vi "AlliGator Build Image Profile Plots.vi"(0 "Intensity":dbl[](array[numeric]), 1 "ROI Type":T4, 2 "Box Profile Type":T3, 3 "ROI Size String":string, 5 "Phase Lifetime":dbl[](array[numeric]), 7 "Average Lifetime/Phasor Ratio":dbl[](array[numeric]), 9 "Fit Parameter":dbl[](array[numeric]), 11 "Error In":errorcluster, 12 "Fit Parameter Name":string, 13 "ratio(T)/<tau>(F)":bool, 14 "< t>_I (F)/<t>_A":bool) -> (4 "Plot Array":T1[](array[typedef]), 15 "Error Out":errorcluster)   [LabVIEW 2021, in "AlliGator Image Profile Window.lvlib"]
doc: "Builds the array of displayed profiles according to the user-selected options and ROI type."
uses:
  AlliGator Image Profile Window.lvlib
  Image/Image ROI Type.ctl
  Image/Box Profile Type.ctl
  AlliGator Image Profile Plot Data.ctl
  Graphs/XY Graph/XY Plot Data.ctl
  Arrays/Linear Ramp End Options.ctl
  52adedef-4fce-46da-a191-00be4efc5a4e.vi
  7c534c3e-da10-41db-a8ff-5ea6a11f1b7c.vi
  c62035f1-53a3-4edf-964a-62b160a8d83f.vi
  258de3ba-5316-44aa-b6b1-8f05b3134f67.vi
  Graphs/XY Graph/XY Graph Add-Ons.lvlib
  Arrays/Arrays.lvlib
  Image/Image.lvlib
panel:
  # "see the AlliGator License on the block diagram (Ctrl+E or Window:Show Block Diagram)"
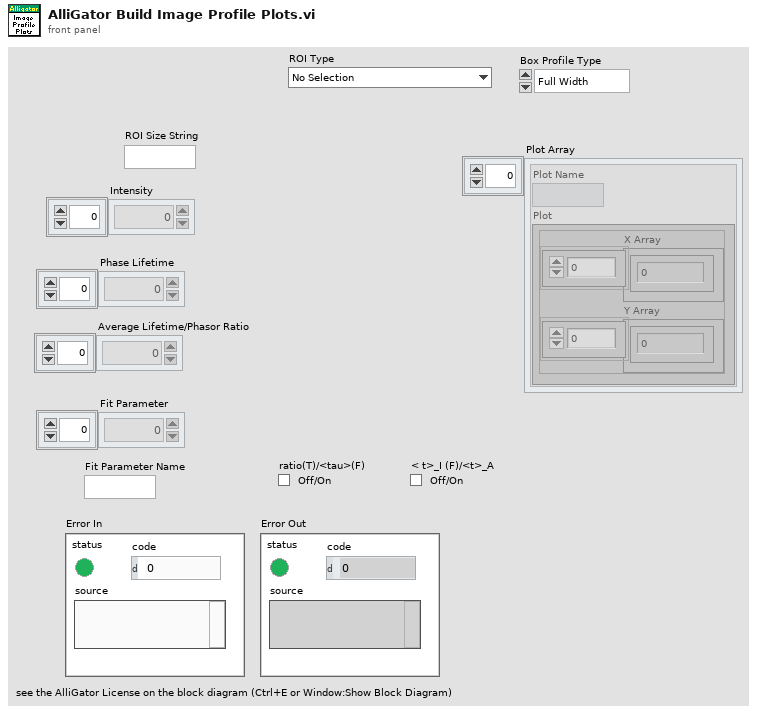
[diagram p1: front panel]
types:
  T1 = typedef "AlliGator Image Profile Window.lvlib/AlliGator Image Profile Plot Data.ctl" = cluster{"Plot Name":string, "Plot":T2}
  T2 = typedef "XY Graph Add-Ons.lvlib/XY Plot Data.ctl" = cluster{"X Array":dbl[], "Y Array":dbl[]}
  T3 = typedef "Image.lvlib/Box Profile Type.ctl" = enum16{"Full Width", "Half Width"}
  T4 = typedef "Image.lvlib/Image ROI Type.ctl" = enum16{"No Selection", "Point", "Line", "Rectangle", "Oval", "Polygon", "Freehand Region", "Annulus", "Unused2", "Unused3", "Broken Line", "Freehand Line", "Rotated Rectangle"}
  T5 = typedef "Arrays.lvlib/Linear Ramp End Options.ctl" = enum16{"Include Min/Exclude Max", "Exclude Min/Include Max", "Include Both Ends", "Exclude Both Ends"}
  T6 = cluster{"Ramp":dbl[], "Average Lifetime/Phasor Ratio":dbl[]}
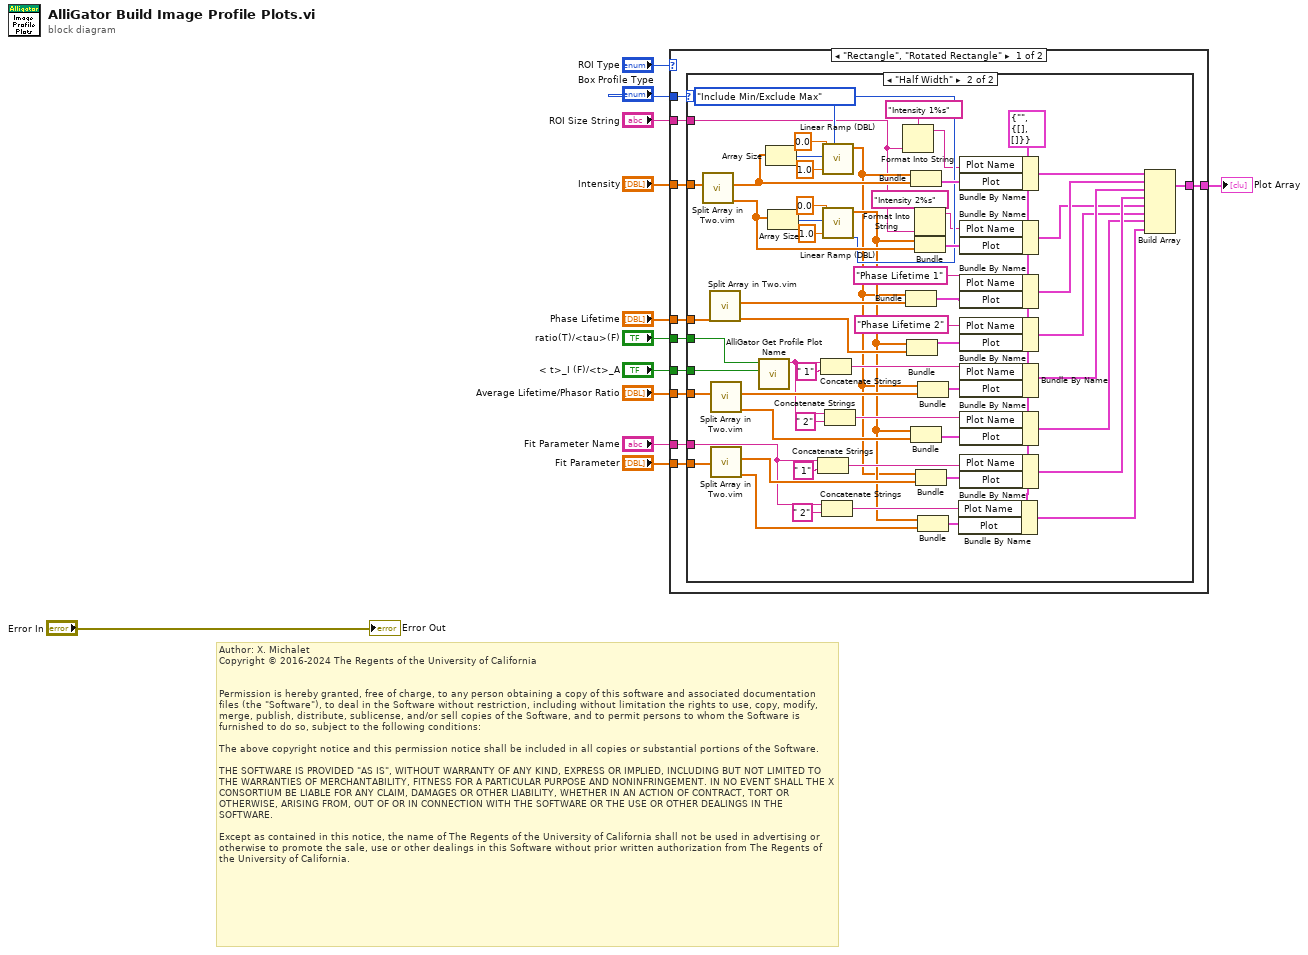
[diagram p0: block diagram]
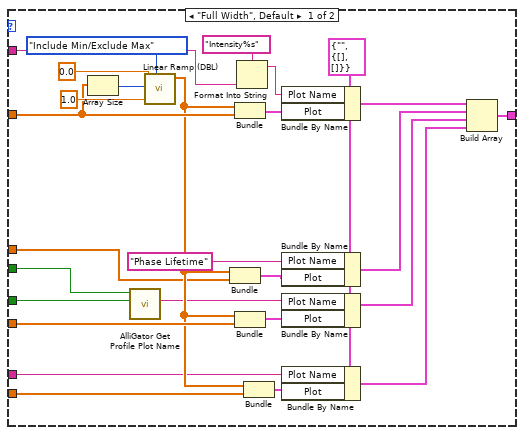
[diagram p2: hidden frame]
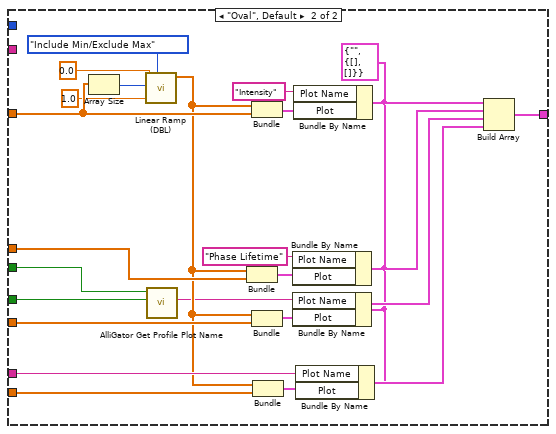
[diagram p3: hidden frame]
diagram:
  # "Author: X. Michalet\nCopyright © 2016-2024 The Regents of the University of California\n \n\nPermission is hereby granted, free of charge, to any person obtaining a copy of this software and associated documentation files (the \"Software\"), to deal in the Software without restriction, including without limitation the rights to use, copy, modify, merge, publish, distribute, sublicense, and/or sell copies of the Software, and to permit persons to whom the Software is furnished to do so, subject to the following conditions:\n\nThe above copyright notice and this permission notice shall be included in all copies or substantial portions of the Software.\n\nTHE SOFTWARE IS PROVIDED \"AS IS\", WITHOUT WARRANTY OF ANY KIND, EXPRESS OR IMPLIED, INCLUDING BUT NOT LIMITED TO THE WARRANTIES OF MERCHANTABILITY, FITNESS FOR A PARTICULAR PURPOSE AND NONINFRINGEMENT. IN NO EVENT SHALL THE X CONSORTIUM BE LIABLE FOR ANY CLAIM, DAMAGES OR OTHER LIABILITY, WHETHER IN AN ACTION OF CONTRACT, TORT OR OTHERWISE, ARISING FROM, OUT OF OR IN CONNECTION WITH THE SOFTWARE OR THE USE OR OTHER DEALINGS IN THE SOFTWARE.\n\nExcept as contained in this notice, the name of The Regents of the University of California shall not be used in advertising or otherwise to promote the sale, use or other dealings in this Software without prior written authorization from The Regents of the University of California."
  n1 = case shown="\"Rectangle\", \"Rotated Rectangle\"" "ROI Type" {
    tunnel: [w22 w132] -> w3
    tunnel: "Intensity" -> [w21 w131]
    tunnel: "Average Lifetime/Phasor Ratio" -> [w20 w130]
    tunnel: "Fit Parameter" -> [w19 w129]
    tunnel: "Fit Parameter Name" -> [w18 w128]
    tunnel: "< t>_I (F)/<t>_A" -> [w17 w127]
    tunnel: "ratio(T)/<tau>(F)" -> [w16 w126]
    tunnel: "Phase Lifetime" -> [w15 w125]
    tunnel: "Box Profile Type" -> [w14 _]
    tunnel: "ROI Size String" -> [w13 _]
    frame "Rectangle", "Rotated Rectangle" {
      n2 = case shown="\"Half Width\"" w14 {
        tunnel: [w43 w101] -> w22
        tunnel: w21 -> [w42 w91]
        tunnel: w20 -> [w38 w76]
        tunnel: w19 -> [w35 w63]
        tunnel: w18 -> [w30 w59]
        tunnel: w17 -> [w28 w93]
        tunnel: w16 -> [w27 w92]
        tunnel: w15 -> [w26 w81]
        tunnel: w13 -> [w23 w50]
        frame "Full Width", Default {
          w31 = T1 {"Plot Name"="", "Plot"={"X Array"=[], "Y Array"=[]}} ("Plot Data")
          n3 = Array Size(array=w42) -> (size(s)=w46:i32)
          n4 = call "AlliGator Get Profile Plot Name.vi"("I-weighted (F)/A=weighted"=w28, "ratio(T)/<tau>(F)"=w27) -> ("Plot Name Suffix"=w29:string)  [unwired: 9 in]
          n5 = call "Linear Ramp (DBL).vi"("Options"=Linear_Ramp_End_Options."Include Min/Exclude Max", "Delta"=1.0, "Max"=w46, "Min"=0.0) -> ("Ramp"=w34:dbl[])  [unwired: 6 in, 1 out]
          n6 = Bundle("Ramp"=w34, "Phase Lifetime"=w26) -> (w41:cluster{"Ramp":dbl[], "Phase Lifetime":dbl[]})  [unwired: 1 in]
          n7 = Bundle("Ramp"=w34, "Intensity"=w42) -> (w45:cluster{"Ramp":dbl[], "Intensity":dbl[]})  [unwired: 1 in]
          n8 = Bundle("Ramp"=w34, "Average Lifetime/Phasor Ratio"=w38) -> (w37:T6)  [unwired: 1 in]
          n9 = Format Into String(format string="Intensity%s" ("Plot Name"), w23) -> (resulting string=w24:string)  [unwired: 2 in, 1 out]
          n10 = Bundle("Ramp"=w34, "Fit Parameter"=w35) -> (w33:cluster{"Ramp":dbl[], "Fit Parameter":dbl[]})  [unwired: 1 in]
          n11 = Bundle By Name(cluster=w31, "Plot Name"=w24, "Plot"=w45) -> (w44:T1)
          n12 = Bundle By Name(cluster=w31, "Plot Name"="Phase Lifetime", "Plot"=w41) -> (w39:T1)
          n13 = Bundle By Name(cluster=w31, "Plot Name"=w29, "Plot"=w37) -> (w36:T1)
          n14 = Bundle By Name(cluster=w31, "Plot Name"=w30, "Plot"=w33) -> (w32:T1)
          n15 = Build Array(w44, w39, w36, w32) -> (w43:T1[])
        }
        frame "Half Width" {
          w84 = Linear_Ramp_End_Options."Include Min/Exclude Max" ("Options")
          w61 = T1 {"Plot Name"="", "Plot"={"X Array"=[], "Y Array"=[]}} ("Plot Data")
          n16 = call "Split Array in Two.vim"("Array in"=w91) -> ("Second Half Array"=w85:dbl[], "First Half Array"=w90:dbl[])  [unwired: 9 in]
          n17 = call "Split Array in Two.vim"("Array in"=w81) -> ("Second Half Array"=w79:dbl[], "First Half Array"=w80:dbl[])  [unwired: 9 in]
          n18 = call "Split Array in Two.vim"("Array in"=w76) -> ("Second Half Array"=w73:dbl[], "First Half Array"=w75:dbl[])  [unwired: 9 in]
          n19 = call "Split Array in Two.vim"("Array in"=w63) -> ("Second Half Array"=w55:dbl[], "First Half Array"=w64:dbl[])  [unwired: 9 in]
          n20 = call "AlliGator Get Profile Plot Name.vi"("I-weighted (F)/A=weighted"=w93, "ratio(T)/<tau>(F)"=w92) -> ("Plot Name Suffix"=w69:string)  [unwired: 9 in]
          n21 = Array Size(array=w90) -> (size(s)=w105:i32)
          n22 = Array Size(array=w85) -> (size(s)=w88:i32)
          n23 = Concatenate Strings(w59, " 1" ("string")) -> (w65:string)
          n24 = Concatenate Strings(w69, " 1" ("string")) -> (w72:string)
          n25 = Concatenate Strings(w59, " 2" ("string")) -> (w60:string)
          n26 = call "Linear Ramp (DBL).vi"("Options"=w84, "Delta"=1.0, "Max"=w105, "Min"=0.0) -> ("Ramp"=w54:dbl[])  [unwired: 6 in, 1 out]
          n27 = call "Linear Ramp (DBL).vi"("Options"=w84, "Delta"=1.0, "Max"=w88, "Min"=0.0) -> ("Ramp"=w57:dbl[])  [unwired: 6 in, 1 out]
          n28 = Concatenate Strings(w69, " 2" ("string")) -> (w68:string)
          n29 = Format Into String(format string="Intensity 1%s" ("Plot Name"), w50) -> (resulting string=w53:string)  [unwired: 2 in, 1 out]
          n30 = Bundle("Ramp"=w54, "First Half Array"=w80) -> (w100:cluster{"Ramp":dbl[], "First Half Array":dbl[]})  [unwired: 1 in]
          n31 = Bundle("Ramp"=w57, "Second Half Array"=w79) -> (w78:cluster{"Ramp":dbl[], "Second Half Array":dbl[]})  [unwired: 1 in]
          n32 = Bundle("Ramp"=w54, "First Half Array"=w90) -> (w104:cluster{"Ramp":dbl[], "First Half Array":dbl[]})  [unwired: 1 in]
          n33 = Bundle("Ramp"=w57, "Second Half Array"=w73) -> (w74:cluster{"Ramp":dbl[], "Second Half Array":dbl[]})  [unwired: 1 in]
          n34 = Format Into String(format string="Intensity 2%s" ("Plot Name"), w50) -> (resulting string=w51:string)  [unwired: 2 in, 1 out]
          n35 = Bundle("Ramp"=w57, "Second Half Array"=w85) -> (w89:cluster{"Ramp":dbl[], "Second Half Array":dbl[]})  [unwired: 1 in]
          n36 = Bundle("Ramp"=w54, "First Half Array"=w64) -> (w95:cluster{"Ramp":dbl[], "First Half Array":dbl[]})  [unwired: 1 in]
          n37 = Bundle("Ramp"=w54, "First Half Array"=w75) -> (w97:cluster{"Ramp":dbl[], "First Half Array":dbl[]})  [unwired: 1 in]
          n38 = Bundle("Ramp"=w57, "Second Half Array"=w55) -> (w62:cluster{"Ramp":dbl[], "Second Half Array":dbl[]})  [unwired: 1 in]
          n39 = Bundle By Name(cluster=w61, "Plot Name"=w60, "Plot"=w62) -> (w56:T1)
          n40 = Bundle By Name(cluster=w61, "Plot Name"=w53, "Plot"=w104) -> (w102:T1)
          n41 = Bundle By Name(cluster=w61, "Plot Name"=w51, "Plot"=w89) -> (w83:T1)
          n42 = Bundle By Name(cluster=w61, "Plot Name"="Phase Lifetime 1", "Plot"=w100) -> (w98:T1)
          n43 = Bundle By Name(cluster=w61, "Plot Name"="Phase Lifetime 2", "Plot"=w78) -> (w77:T1)
          n44 = Bundle By Name(cluster=w61, "Plot Name"=w72, "Plot"=w97) -> (w96:T1)
          n45 = Bundle By Name(cluster=w61, "Plot Name"=w68, "Plot"=w74) -> (w67:T1)
          n46 = Bundle By Name(cluster=w61, "Plot Name"=w65, "Plot"=w95) -> (w94:T1)
          n47 = Build Array(w102, w98, w96, w94, w83, w77, w67, w56) -> (w101:T1[])
        }
      }
    }
    frame "Oval", Default {
      w109 = T1 {"Plot Name"="", "Plot"={"X Array"=[], "Y Array"=[]}} ("Plot Data")
      n48 = Array Size(array=w131) -> (size(s)=w121:i32)
      n49 = call "Linear Ramp (DBL).vi"("Options"=Linear_Ramp_End_Options."Include Min/Exclude Max", "Delta"=1.0, "Max"=w121, "Min"=0.0) -> ("Ramp"=w112:dbl[])  [unwired: 6 in, 1 out]
      n50 = call "AlliGator Get Profile Plot Name.vi"("I-weighted (F)/A=weighted"=w127, "ratio(T)/<tau>(F)"=w126) -> ("Plot Name Suffix"=w108:string)  [unwired: 9 in]
      n51 = Bundle("Ramp"=w112, "Phase Lifetime"=w125) -> (w117:cluster{"Ramp":dbl[], "Phase Lifetime":dbl[]})  [unwired: 1 in]
      n52 = Bundle("Ramp"=w112, "Intensity"=w131) -> (w120:cluster{"Ramp":dbl[], "Intensity":dbl[]})  [unwired: 1 in]
      n53 = Bundle("Ramp"=w112, "Average Lifetime/Phasor Ratio"=w130) -> (w114:T6)  [unwired: 1 in]
      n54 = Bundle("Ramp"=w112, "Fit Parameter"=w129) -> (w111:cluster{"Ramp":dbl[], "Fit Parameter":dbl[]})  [unwired: 1 in]
      n55 = Bundle By Name(cluster=w109, "Plot Name"="Phase Lifetime", "Plot"=w117) -> (w115:T1)
      n56 = Bundle By Name(cluster=w109, "Plot Name"=w108, "Plot"=w114) -> (w113:T1)
      n57 = Bundle By Name(cluster=w109, "Plot Name"="Intensity", "Plot"=w120) -> (w118:T1)
      n58 = Bundle By Name(cluster=w109, "Plot Name"=w128, "Plot"=w111) -> (w110:T1)
      n59 = Build Array(w118, w115, w113, w110) -> (w132:T1[])
    }
  }
  "Plot Array" <- w3
  "Error Out" <- "Error In"
